vi "isSessionPresent.vi"(8 "error in":errorcluster, 10 "Client ID":string, 11 "Server in":refnum<class "Server.lvclass">) -> (0 "error out":errorcluster, 1 "Session Present":bool, 2 "Client ID dup":string, 3 "Server out":refnum<class "Server.lvclass">)   [LabVIEW 2013, in "MQTT Server.lvlib" / "Server.lvclass"]
uses:
  Server.lvclass
  Session/Session State -- cluster.ctl
  StoredSessions/StoredSessions.lvclass
  Session/Session.lvclass
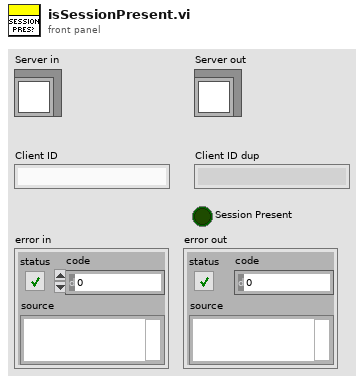
[diagram p1: front panel]
types:
  T1 = typedef "MQTT Server.lvlib/Session.lvclass/Session State -- cluster.ctl" = cluster{"CleanSession":bool, "Client ID":string}
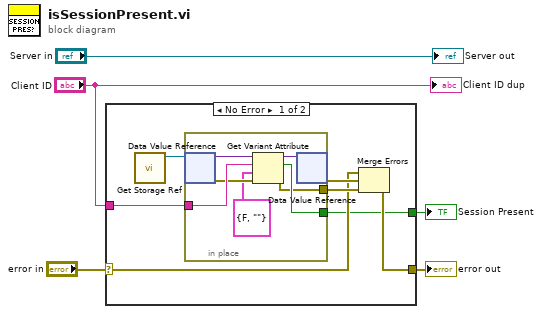
[diagram p0: block diagram]
diagram:
  n1 = case shown="No Error" "error in" {
    selector: "error in" -> [w8 w20]
    tunnel: [w7 w20] -> w4
    tunnel: "Client ID" -> [w11 _]
    tunnel: [w6 _] -> w3
    frame No Error {
      n2 = call "Get Storage Ref.vi"() -> ("Storage"=w12:refnum<data-value>)  [unwired: 11 in]
      n3 = in-place {
        in-place-border: w11 -> [w18]
        in-place-border: [w13] -> w10
        in-place-border: [w15] -> w6
        n4 = in-place-dvr #1(w12) -> (w19:variant, w16:errorcluster)
        n5 = Get Variant Attribute(Variant=w19, name=w18, default value (empty Variant)=T1 {"CleanSession"=FALSE, "Client ID"=""} ("Session State"), error in=w16) -> (duplicate Variant=w17:variant, found=w15:bool, error out=w13:errorcluster)  [unwired: 1 out]
        n6 = in-place-dvr #1(w17) -> (w9:errorcluster)  [unwired: 1 out]
      }
      n7 = Merge Errors(w8, w9, w10) -> (w7:errorcluster)
    }
    frame Error {
    }
  }
  "error out" <- w4
  "Session Present" <- w3
  "Client ID dup" <- "Client ID"
  "Server out" <- "Server in"
